vi "LABVIEW PRATICA 7 ATV2.vi"() -> ()   [LabVIEW 2017]
uses:
  <vilib>/platform/TimedLoop/XDataNode/XDataNode.xnode
  <vilib>/Platform/TimedLoop/XDataNode/nitl_modes.ctl
  <vilib>/Platform/TimedLoop/XDataNode/XDNodeRunTimeDep.lvlib
  <vilib>/Platform/TimedLoop/XDataNode/wakeup.ctl
  <vilib>/Platform/TimedLoop/XDataNode/timing_clust.ctl
panel:
  in  "stop":bool
  out "Waveform Chart":dbl(graph)
  in  "Ki":dbl
  in  "Kp":dbl
  in  "Set-point":dbl
  out "Tensão Bomba":dbl
  out "Nível(mm)":dbl
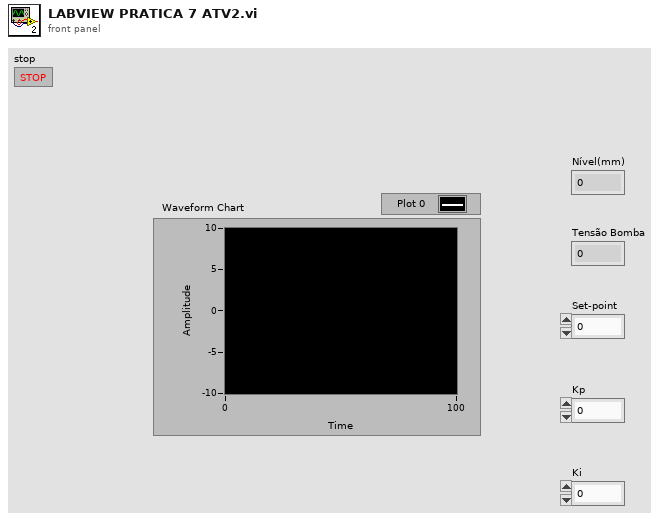
[diagram p1: front panel]
types:
  T1 = typedef "XDNodeRunTimeDep.lvlib/timing_clust.ctl" = cluster{"Expected End [f-1]":u64, "Actual End [f-1]":u64, "Finished Late? [f-1]":bool, "Expected End [i-1]":u64, "Actual End [i-1]":u64, "Finished Late? [i-1]":bool, "Expected Start [i]":u64, "Actual Start [i]":u64, "Expected Start [f]":u64, "Actual Start [f]":u64, "Source Name":string, "Structure Name":string, "Period":i64, "Deadline":i64, "Offset":i64, "Start":i64, "Priority":i32, "Timeout":i32, "Mode":T2, "Wakeup Reason":T3, "Error":errorcluster, "Source Type":string, "Secondary Source Type":string, "Global End Time":u64, "Global Start Time":u64, "Frame Duration":u64, "Iteration Duration":u64, "Assigned CPU":i32, "I/O Scan Engine Mode":u32}
  T2 = typedef "XDNodeRunTimeDep.lvlib/nitl_modes.ctl" = enum32{"No Change", "Process missed periods, maintain original phase", "Discard missed periods, maintain original phase", "Process missed periods, ignore original phase", "Discard missed periods, ignore original phase"}
  T3 = typedef "XDNodeRunTimeDep.lvlib/wakeup.ctl" = enum32{"Normal", "Aborted", "Asynchronous wakeup", "Timing source error", "Timed loop error", "Timeout"}
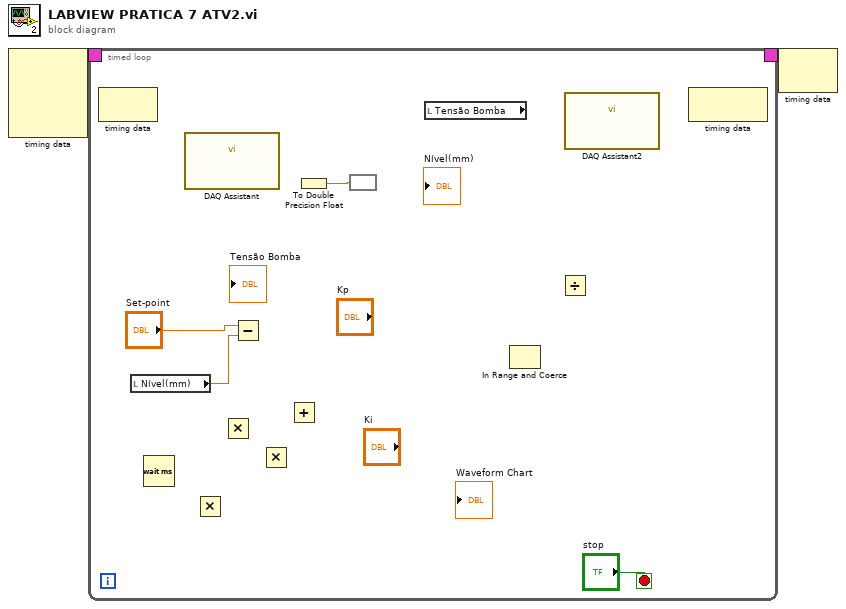
[diagram p0: block diagram]
diagram:
  n1 = node-c288() -> (w2:T1)  [unwired: 4 in]
  n2 = timed-loop {
    timing: w2 -> [_]
    timing-out: [_] -> w1
    stop <- "stop" stop-if-true
    n3 = node-c288() -> ()  [unwired: 1 in, 1 out]
    n4 = local read "Nível(mm)"() -> (w4:dbl)
    n5 = Wait (ms)() -> ()  [unwired: 1 in, 1 out]
    n6 = call "DAQ Assistant"() -> ()  [unwired: 12 in]
    n7 = Multiply() -> ()  [unwired: 2 in, 1 out]
    n8 = Multiply() -> ()  [unwired: 2 in, 1 out]
    n9 = Subtract(x="Set-point", y=w4) -> ()  [unwired: 1 out]
    n10 = Multiply() -> ()  [unwired: 2 in, 1 out]
    n11 = Add() -> ()  [unwired: 2 in, 1 out]
    n12 = To Double Precision Float() -> (double precision float=w3:dbl)  [unwired: 1 in]
    n13 = expression code=""(w3) -> ()  [unwired: 1 out]
    n14 = local read "Tensão Bomba"() -> ()  [unwired: 1 out]
    n15 = In Range and Coerce() -> ()  [unwired: 3 in, 2 out]
    n16 = Divide() -> ()  [unwired: 2 in, 1 out]
    n17 = call "DAQ Assistant2"() -> ()  [unwired: 12 in]
    n18 = node-c288() -> ()  [unwired: 1 in, 1 out]
  }
  n19 = node-c288(w1) -> ()  [unwired: 1 out]
